vi "GetInclinometerDataField.vi"(10 "Telemetry Data":string, 11 "Cluster in":refnum<vi>) -> (3 "Array":string[](array[string]))   [LabVIEW 2016]
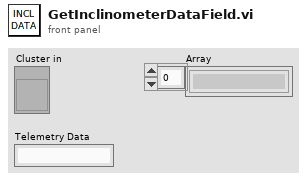
[diagram p1: front panel]
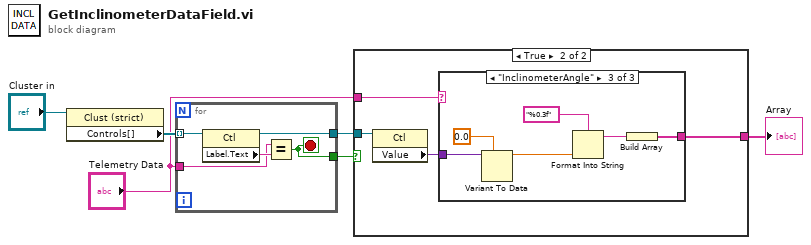
[diagram p0: block diagram]
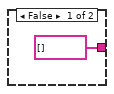
[diagram p2: hidden frame]
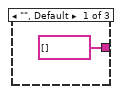
[diagram p3: hidden frame]
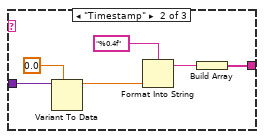
[diagram p4: hidden frame]
diagram:
  n1 = property on="Property Node" class="Clust (strict)"(reference="Cluster in") -> ("Controls[]"=w5:refnum<vi>[])  [unwired: 1 in, 2 out]
  n2 = for {
    tunnel: w5 -> [w11] mode=indexing
    tunnel: [w10] -> w2
    tunnel: "Telemetry Data" -> [w8]
    tunnel: [w7] -> w1
    stop <- w7 stop-if-true
    n3 = property on="Property Node" class="Ctl"(reference=w11) -> (reference out=w10:refnum<vi>, "Label.Text"=w9:string)  [unwired: 1 in, 1 out]
    n4 = Equal?(x=w8, y=w9) -> (x = y?=w7:bool)
  }
  n5 = case shown="True" w1 {
    tunnel: "Telemetry Data" -> [_ w16]
    tunnel: w2 -> [_ w15]
    tunnel: [string[] [] w13] -> w6
    frame False {
    }
    frame True {
      n6 = property on="Property Node" class="Ctl"(reference=w15) -> ("Value"=w14:variant)  [unwired: 1 in, 2 out]
      n7 = case shown="\"InclinometerAngle\"" w16 {
        tunnel: [string[] [] w21 w27] -> w13
        tunnel: w14 -> [_ w19 w25]
        frame "", Default {
        }
        frame "Timestamp" {
          n8 = Variant To Data(type=0.0, Variant=w19) -> (data=w20:dbl)  [unwired: 1 in, 1 out]
          n9 = Format Into String(format string="%0.4f", w20) -> (resulting string=w22:string)  [unwired: 2 in, 1 out]
          n10 = Build Array(w22) -> (w21:string[])
        }
        frame "InclinometerAngle" {
          n11 = Variant To Data(type=0.0, Variant=w25) -> (data=w26:dbl)  [unwired: 1 in, 1 out]
          n12 = Format Into String(format string="%0.3f", w26) -> (resulting string=w28:string)  [unwired: 2 in, 1 out]
          n13 = Build Array(w28) -> (w27:string[])
        }
      }
    }
  }
  "Array" <- w6
